vi "ip.vi"(1 "Set":T2, 2 "T":bool, 3 "R":bool) -> (0 "com_number":T1)   [LabVIEW 2013]
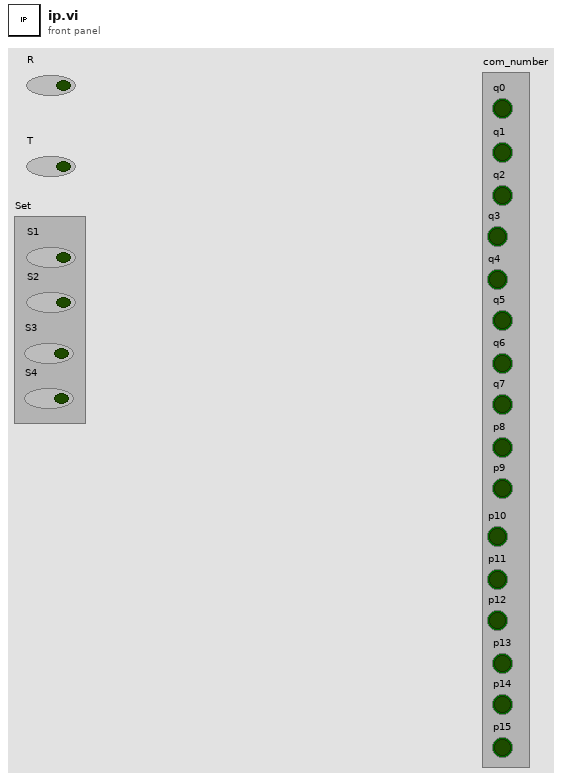
[diagram p1: front panel]
types:
  T1 = cluster{"q0":bool, "q1":bool, "q2":bool, "q3":bool, "q4":bool, "q5":bool, "q6":bool, "q7":bool, "p8":bool, "p9":bool, "p10":bool, "p11":bool, "p12":bool, "p13":bool, "p14":bool, "p15":bool}
  T2 = cluster{"S1":bool, "S2":bool, "S3":bool, "S4":bool}
  T3 = cluster{bool, bool, bool, bool, bool, bool, bool, bool, bool, bool, bool, bool, bool, bool, bool, bool}
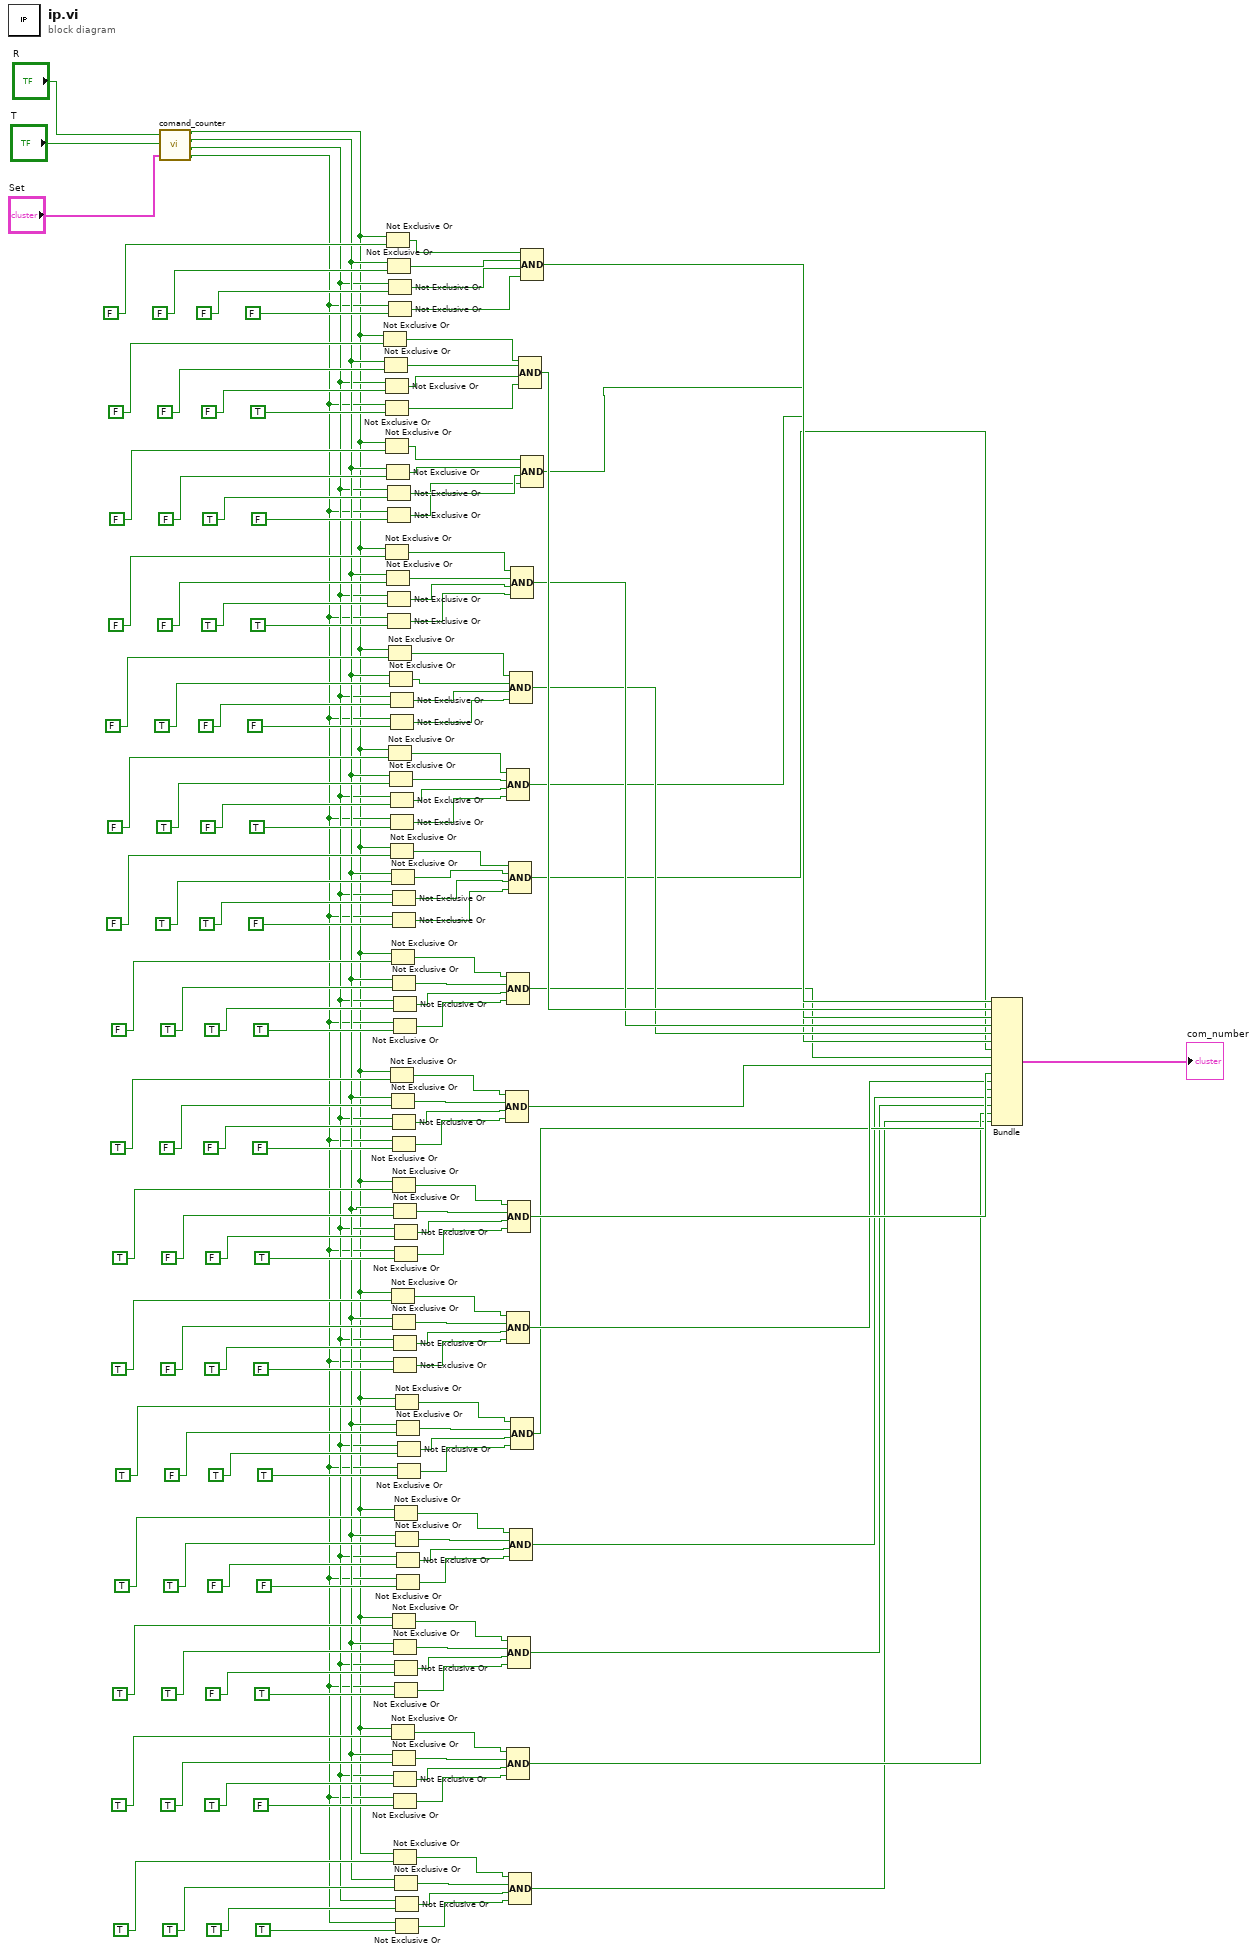
[diagram p0: block diagram]
diagram:
  n1 = call "comand_counter.vi"("R"="R", "такты"="T", "Set"="Set") -> ("q4"=w1:bool, "q3"=w12:bool, "q2"=w11:bool, "q1"=w10:bool)
  n2 = Not Exclusive Or(1:FALSE, 2:w1) -> (0:w116:bool)
  n3 = Not Exclusive Or(1:FALSE, 2:w12) -> (0:w115:bool)
  n4 = Not Exclusive Or(1:FALSE, 2:w11) -> (0:w114:bool)
  n5 = Not Exclusive Or(1:TRUE, 2:w10) -> (0:w113:bool)
  n6 = Not Exclusive Or(1:FALSE, 2:w1) -> (0:w112:bool)
  n7 = Not Exclusive Or(1:FALSE, 2:w1) -> (0:w108:bool)
  n8 = Not Exclusive Or(1:FALSE, 2:w1) -> (0:w120:bool)
  n9 = Not Exclusive Or(1:FALSE, 2:w12) -> (0:w111:bool)
  n10 = Not Exclusive Or(1:FALSE, 2:w12) -> (0:w107:bool)
  n11 = Not Exclusive Or(1:FALSE, 2:w12) -> (0:w119:bool)
  n12 = Not Exclusive Or(1:TRUE, 2:w11) -> (0:w110:bool)
  n13 = Not Exclusive Or(1:FALSE, 2:w10) -> (0:w109:bool)
  n14 = Not Exclusive Or(1:TRUE, 2:w11) -> (0:w106:bool)
  n15 = Not Exclusive Or(1:TRUE, 2:w10) -> (0:w105:bool)
  n16 = Not Exclusive Or(1:FALSE, 2:w11) -> (0:w118:bool)
  n17 = Not Exclusive Or(1:FALSE, 2:w10) -> (0:w117:bool)
  n18 = Not Exclusive Or(1:FALSE, 2:w1) -> (0:w104:bool)
  n19 = Not Exclusive Or(1:FALSE, 2:w1) -> (0:w100:bool)
  n20 = Not Exclusive Or(1:TRUE, 2:w12) -> (0:w103:bool)
  n21 = Not Exclusive Or(1:TRUE, 2:w12) -> (0:w99:bool)
  n22 = Not Exclusive Or(1:FALSE, 2:w11) -> (0:w102:bool)
  n23 = Not Exclusive Or(1:FALSE, 2:w10) -> (0:w101:bool)
  n24 = Not Exclusive Or(1:FALSE, 2:w11) -> (0:w98:bool)
  n25 = Not Exclusive Or(1:TRUE, 2:w10) -> (0:w97:bool)
  n26 = Not Exclusive Or(1:FALSE, 2:w1) -> (0:w96:bool)
  n27 = Not Exclusive Or(1:TRUE, 2:w1) -> (0:w72:bool)
  n28 = Not Exclusive Or(1:TRUE, 2:w12) -> (0:w95:bool)
  n29 = Not Exclusive Or(1:FALSE, 2:w1) -> (0:w92:bool)
  n30 = Not Exclusive Or(1:FALSE, 2:w12) -> (0:w71:bool)
  n31 = Not Exclusive Or(1:TRUE, 2:w1) -> (0:w56:bool)
  n32 = Not Exclusive Or(1:TRUE, 2:w1) -> (0:w24:bool)
  n33 = Not Exclusive Or(1:TRUE, 2:w11) -> (0:w94:bool)
  n34 = Not Exclusive Or(1:FALSE, 2:w10) -> (0:w93:bool)
  n35 = Not Exclusive Or(1:TRUE, 2:w12) -> (0:w91:bool)
  n36 = Not Exclusive Or(1:FALSE, 2:w11) -> (0:w70:bool)
  n37 = Not Exclusive Or(1:FALSE, 2:w10) -> (0:w69:bool)
  n38 = Not Exclusive Or(1:TRUE, 2:w1) -> (0:w64:bool)
  n39 = Not Exclusive Or(1:FALSE, 2:w12) -> (0:w55:bool)
  n40 = Not Exclusive Or(1:TRUE, 2:w1) -> (0:w32:bool)
  n41 = Not Exclusive Or(1:TRUE, 2:w12) -> (0:w23:bool)
  n42 = Not Exclusive Or(1:TRUE, 2:w11) -> (0:w90:bool)
  n43 = Not Exclusive Or(1:TRUE, 2:w10) -> (0:w89:bool)
  n44 = Not Exclusive Or(1:FALSE, 2:w12) -> (0:w63:bool)
  n45 = Not Exclusive Or(1:TRUE, 2:w11) -> (0:w54:bool)
  n46 = Not Exclusive Or(1:FALSE, 2:w10) -> (0:w53:bool)
  n47 = Not Exclusive Or(1:TRUE, 2:w12) -> (0:w31:bool)
  n48 = Not Exclusive Or(1:TRUE, 2:w11) -> (0:w22:bool)
  n49 = Not Exclusive Or(1:FALSE, 2:w10) -> (0:w21:bool)
  n50 = Not Exclusive Or(1:TRUE, 2:w1) -> (0:w16:bool)
  n51 = Not Exclusive Or(1:FALSE, 2:w11) -> (0:w62:bool)
  n52 = Not Exclusive Or(1:TRUE, 2:w10) -> (0:w61:bool)
  n53 = Not Exclusive Or(1:TRUE, 2:w1) -> (0:w40:bool)
  n54 = Not Exclusive Or(1:FALSE, 2:w11) -> (0:w30:bool)
  n55 = Not Exclusive Or(1:TRUE, 2:w10) -> (0:w29:bool)
  n56 = Not Exclusive Or(1:TRUE, 2:w12) -> (0:w15:bool)
  n57 = Not Exclusive Or(1:TRUE, 2:w1) -> (0:w48:bool)
  n58 = Not Exclusive Or(1:TRUE, 2:w12) -> (0:w39:bool)
  n59 = Not Exclusive Or(1:TRUE, 2:w11) -> (0:w14:bool)
  n60 = Not Exclusive Or(1:TRUE, 2:w10) -> (0:w13:bool)
  n61 = Not Exclusive Or(1:FALSE, 2:w12) -> (0:w47:bool)
  n62 = Not Exclusive Or(1:FALSE, 2:w11) -> (0:w38:bool)
  n63 = Not Exclusive Or(1:FALSE, 2:w10) -> (0:w37:bool)
  n64 = Not Exclusive Or(1:TRUE, 2:w11) -> (0:w46:bool)
  n65 = Not Exclusive Or(1:TRUE, 2:w10) -> (0:w45:bool)
  n66 = Compound Arithmetic op=AND(w72, w71, w70, w69) -> (w9:bool)
  n67 = Compound Arithmetic op=AND(w100, w99, w98, w97) -> (w80:bool)
  n68 = Compound Arithmetic op=AND(w92, w91, w90, w89) -> (w78:bool)
  n69 = Compound Arithmetic op=AND(w56, w55, w54, w53) -> (w7:bool)
  n70 = Compound Arithmetic op=AND(w24, w23, w22, w21) -> (w3:bool)
  n71 = Compound Arithmetic op=AND(w64, w63, w62, w61) -> (w8:bool)
  n72 = Compound Arithmetic op=AND(w32, w31, w30, w29) -> (w4:bool)
  n73 = Compound Arithmetic op=AND(w96, w95, w94, w93) -> (w79:bool)
  n74 = Compound Arithmetic op=AND(w16, w15, w14, w13) -> (w2:bool)
  n75 = Compound Arithmetic op=AND(w104, w103, w102, w101) -> (w81:bool)
  n76 = Compound Arithmetic op=AND(w40, w39, w38, w37) -> (w5:bool)
  n77 = Compound Arithmetic op=AND(w108, w107, w106, w105) -> (w82:bool)
  n78 = Compound Arithmetic op=AND(w48, w47, w46, w45) -> (w6:bool)
  n79 = Compound Arithmetic op=AND(w116, w115, w114, w113) -> (w84:bool)
  n80 = Compound Arithmetic op=AND(w120, w119, w118, w117) -> (w85:bool)
  n81 = Compound Arithmetic op=AND(w112, w111, w110, w109) -> (w83:bool)
  n82 = Bundle(w85, w84, w83, w82, w81, w80, w79, w78, w9, w8, w7, w6, w5, w4, w3, w2) -> (→"com_number":T3)  [unwired: 1 in]
